vi "Read Serial Data.vi"(8 "error in (no error)":errorcluster, 11 "cCRDS Data in":refnum<class "cCRDS Data.lvclass">) -> (0 "error out":errorcluster, 2 "Serial Data":refnum<class "Data.lvclass">[](array[class]), 3 "cCRDS Data out":refnum<class "cCRDS Data.lvclass">)   [LabVIEW 2015, in "cCRDS Data.lvclass"]
uses:
  cCRDS Data.lvclass
  Reusable/Data/Data.lvclass
  cCRDS Data.lvclass/cCRDS Data.ctl
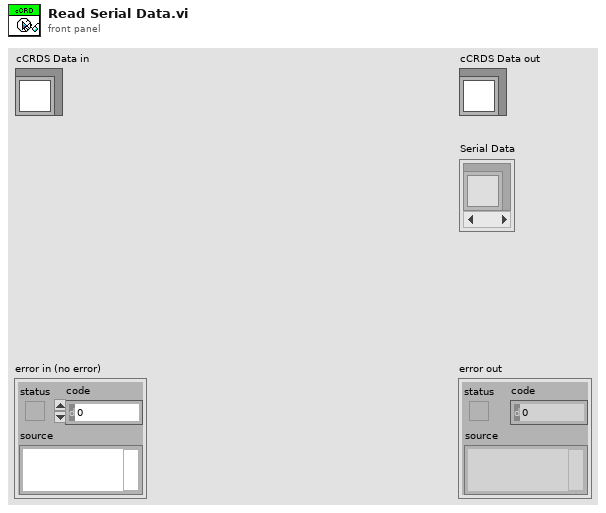
[diagram p1: front panel]
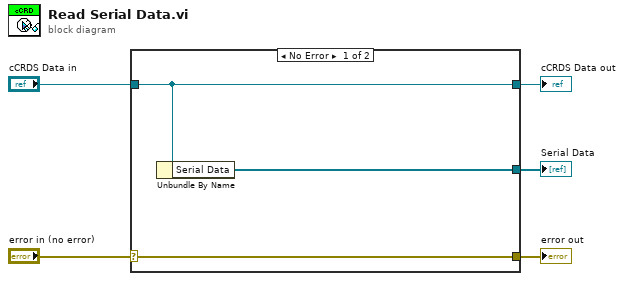
[diagram p0: block diagram]
diagram:
  n1 = case shown="No Error" "error in (no error)" {
    selector: "error in (no error)" -> [w8 w9]
    tunnel: [w8 w9] -> w4
    tunnel: [w7 w10] -> w2
    tunnel: "cCRDS Data in" -> [w7 w10]
    tunnel: [w6 _] -> w1
    frame No Error {
      n2 = Unbundle By Name(w7) -> ("Serial Data"=w6:refnum<class "Data.lvclass">[])
    }
    frame Error {
    }
  }
  "error out" <- w4
  "cCRDS Data out" <- w2
  "Serial Data" <- w1
